vi "point_to_time_4_sin_pulse.vi"(8 "DAC frequency(MHz)":dbl, 9 "point location":i32, 10 "Pulse Width":dbl, 11 "Pulse Center (us)":dbl) -> (0 "dt (us)":dbl, 1 "t_finish":dbl, 2 "t - t_start":dbl, 3 "t inside pulse width":bool, 4 "t":dbl)   [LabVIEW 2016]
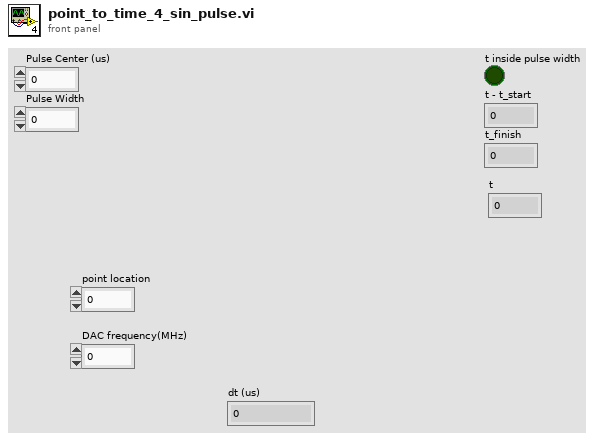
[diagram p1: front panel]
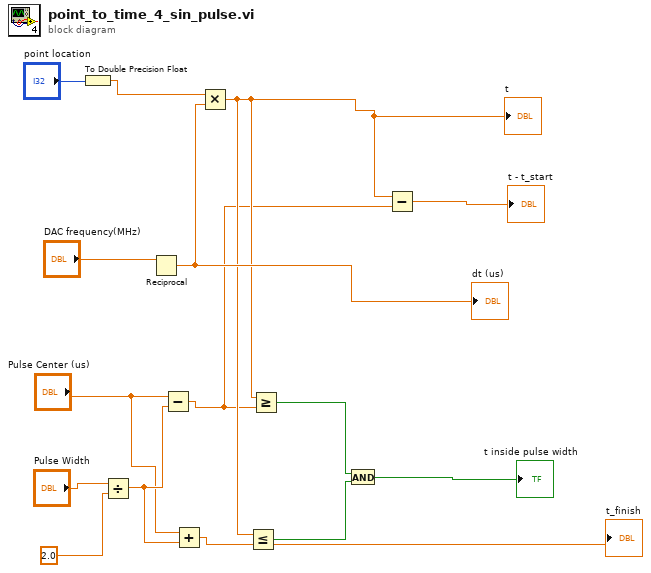
[diagram p0: block diagram]
diagram:
  n1 = To Double Precision Float(number="point location") -> (double precision float=w9:dbl)
  n2 = Divide(x="Pulse Width", y=2.0) -> (x/y=w11:dbl)
  n3 = Reciprocal(x="DAC frequency(MHz)") -> (1/x=w5:dbl)
  "dt (us)" <- w5
  n4 = Subtract(x="Pulse Center (us)", y=w11) -> (x-y=w2:dbl)
  n5 = Add(x="Pulse Center (us)", y=w11) -> (x+y=w4:dbl)
  "t_finish" <- w4
  n6 = Multiply(x=w9, y=w5) -> (x*y=w3:dbl)
  "t" <- w3
  n7 = Less Or Equal?(x=w3, y=w4) -> (x <= y?=w7:bool)
  n8 = Greater Or Equal?(x=w3, y=w2) -> (x >= y?=w8:bool)
  n9 = And(x=w8, y=w7) -> (x .and. y?=→"t inside pulse width":bool)
  n10 = Subtract(x=w3, y=w2) -> (x-y=→"t - t_start":dbl)
